vi "Set Velocity Setpoint.vi"(8 "error in (no error)":errorcluster, 10 "CCW velocity (rad/s)":dbl, 11 "simulated KUKA youBot wheel motor in":refnum<class "NI_Robotics_KUKA youBot Wheel Motor_Sim.lvclass">) -> (0 "error out":errorcluster, 3 "simulated KUKA youBot wheel motor out":refnum<class "NI_Robotics_KUKA youBot Wheel Motor_Sim.lvclass">)   [LabVIEW 2017, in "NI_Robotics_KUKA youBot Host.lvlib" / "NI_Robotics_KUKA youBot Wheel Motor_Sim.lvclass"]
uses:
  <vilib>/robotics/KUKA youBot/Motor/Wheel Motor Sim/NI_Robotics_KUKA youBot Wheel Motor_Sim.lvclass
  <vilib>/robotics/KUKA youBot/Motor/Wheel Motor Sim/NI_Robotics_KUKA youBot Wheel Motor_Sim.lvclass/NI_Robotics_KUKA youBot Wheel Motor_Sim.ctl
  <vilib>/robotics/Simulator/Robot Factory/Motor/ODESimulator_Motor.lvclass
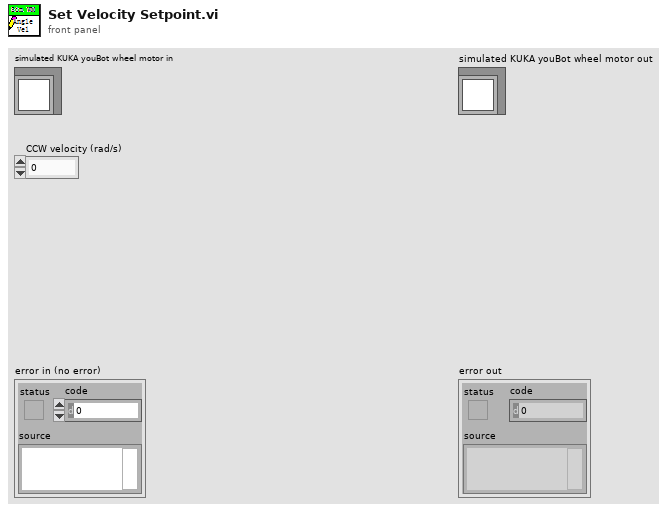
[diagram p1: front panel]
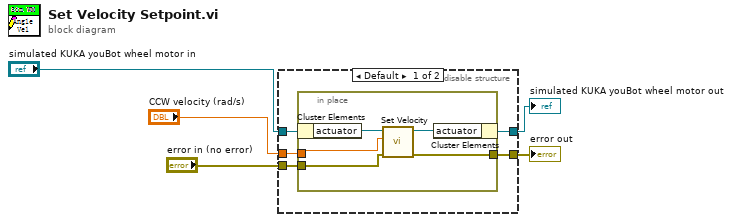
[diagram p0: block diagram]
diagram:
  n1 = disable-structure shown="Default" {
    disable-tunnel: "CCW velocity (rad/s)" -> [w10 _]
    disable-tunnel: "simulated KUKA youBot wheel motor in" -> [w9 w17]
    disable-tunnel: "error in (no error)" -> [w8 w16]
    disable-tunnel: [w7 w16] -> w1
    disable-tunnel: [w6 w17] -> w2
    frame condition #0 (active) {
      n2 = in-place {
        in-place-border: w10 -> [w13]
        in-place-border: w8 -> [w12]
        in-place-border: [w11] -> w7
        n3 = in-place-cluster #1(w9) -> ("actuator"=w15:refnum<class "ODESimulator_Motor.lvclass">)
        n4 = call-dynamic "Set Velocity.vi"("error in (no error)"=w12, "CCW Velocity (0.0 rad/s)"=w13, "Motor in"=w15) -> ("error out"=w11:errorcluster, "Motor out"=w14:refnum<class "ODESimulator_Motor.lvclass">)  [unwired: 7 in]
        n5 = in-place-cluster #1("actuator"=w14) -> (w6:refnum<class "NI_Robotics_KUKA youBot Wheel Motor_Sim.lvclass">)
      }
    }
    frame condition #1 {
    }
  }
  "error out" <- w1
  "simulated KUKA youBot wheel motor out" <- w2
